vi "3.1.vi"(0 "X":dbl) -> (1 "sin(x)":dbl, 2 "cos(x)":dbl)   [LabVIEW 2017]
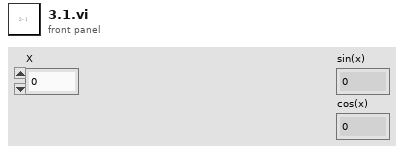
[diagram p1: front panel]
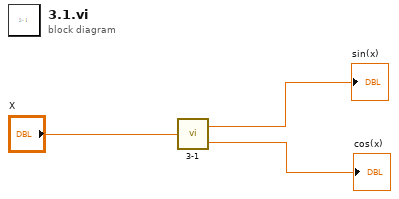
[diagram p0: block diagram]
diagram:
  n1 = call "3-1.vi"("X"="X") -> ("sin(x)"=→"sin(x)":dbl, "cos(x)"=→"cos(x)":dbl)
